vi "DCM System Status.vi"(9 "FIFO Indexes":T4={"System ADC"={"AI 1 [V]"=0, "AI 2 [V]"=0, "AI 3 [V]"=0, "AI 4 [V]"=0, "AI 5 [V]"=0, "AI 6 [V]"=0, "AI 7 [V]"=0, "AI 8 [V]"=0, "AI 9 [V]"=0, "AI 10 [V]"=0, "AI 11 [V]"=0, "AI 12 [V]"=0, "Temp HH 1-6 [C]"=0, "Temp HH 7-12 [C]"=0, "Temp DI A [C]"=0, "Temp DI Zener A [C]"=0, "Temp DI B [C]"=0, "Temp DI Zener B [C]"=0, "Temp CPU [C]"=0, "Temp Fan Intake [C]"=0, "Temp Secondary A [C]"=0, "Temp Primary A [C]"=0, "Temp Boost B [C]"=0, "Primary Range [V]"=0, "Primary A1A2 [V]"=0, "Primary A3A4 [V]"=0, "Primary B3B4 [V]"=0, "Primary B1B2 [V]"=0, "Secondary A1A2 [V]"=0, "Secondary A3A4 [V]"=0, "Secondary B3B4 [V]"=0, "Secondary B1B2 [V]"=0, "Ext HV A [V]"=0, "Ext HV B [V]"=0, "FET Driver [V]"=0, "Fan [V]"=-1, "Battery [V]"=0, "DRVP [V]"=0, "Key [V]"=0, "DI Zener A [V]"=0, "DI Zener B [V]"=0, "Pump Zener A [V]"=0, "Pump Zener B [V]"=0, "MPRD [V]"=0}, "IO Lock"=0, "HH Mode Config Error"=0, "Fan Speed 1 [RPM]"=0, "Fan Speed 2 [RPM]"=0, "Firmware Major Rev"=0, "Firmware Minor Rev"=0, "Internal Fault"=-1, "Fault Value"=-1}, 10 "System State":T1 {"System ADC"."Fan [V]" format="%#_3p"; "System ADC"."Primary B1B2 [V]" format="%#_3p"; "System ADC"."Primary B3B4 [V]" format="%#_3p"; "System ADC"."Primary A3A4 [V]" format="%#_3p"; "System ADC"."Primary A1A2 [V]" format="%#_3p"; "System ADC"."MPRD [V]" format="%#_3p"; "System ADC"."Ext HV B [V]" format="%#_3p"; "System ADC"."Ext HV A [V]" format="%#_3p"; "System ADC"."Pump Zener B [V]" format="%#_3p"; "System ADC"."Pump Zener A [V]" format="%#_3p"; "System ADC"."DI Zener B [V]" format="%#_3p"; "System ADC"."DI Zener A [V]" format="%#_3p"; "System ADC"."Key [V]" format="%#_3p"; "System ADC"."DRVP [V]" format="%#_3p"; "System ADC"."Battery [V]" format="%#_3p"; "System ADC"."FET Driver [V]" format="%#_3p"; "System ADC"."Secondary B1B2 [V]" format="%#_3p"; "System ADC"."Secondary B3B4 [V]" format="%#_3p"; "System ADC"."Secondary A3A4 [V]" format="%#_3p"; "System ADC"."Secondary A1A2 [V]" format="%#_3p"; "System ADC"."Primary Range [V]" format="%#_3p"; "System ADC"."Temp Boost B [C]" format="%#_3p"; "System ADC"."Temp Primary A [C]" format="%#_3p"; "System ADC"."Temp Secondary A [C]" format="%#_3p"; "System ADC"."Temp Fan Intake [C]" format="%#_3p"; "System ADC"."Temp CPU [C]" format="%#_3p"; "System ADC"."Temp DI Zener B [C]" format="%#_3p"; "System ADC"."Temp DI B [C]" format="%#_3p"; "System ADC"."Temp DI Zener A [C]" format="%#_3p"; "System ADC"."Temp DI A [C]" format="%#_3p"; "System ADC"."Temp HH 7-12 [C]" format="%#_3p"; "System ADC"."Temp HH 1-6 [C]" format="%#_3p"; "System ADC"."AI 12 [V]" format="%#_3p"; "System ADC"."AI 11 [V]" format="%#_3p"; "System ADC"."AI 10 [V]" format="%#_3p"; "System ADC"."AI 9 [V]" format="%#_3p"; "System ADC"."AI 8 [V]" format="%#_3p"; "System ADC"."AI 7 [V]" format="%#_3p"; "System ADC"."AI 6 [V]" format="%#_3p"; "System ADC"."AI 5 [V]" format="%#_3p"; "System ADC"."AI 4 [V]" format="%#_3p"; "System ADC"."AI 3 [V]" format="%#_3p"; "System ADC"."AI 2 [V]" format="%#_3p"; "System ADC"."AI 1 [V]" format="%#_3p"}, 11 "Device Outputs in":dbl[](array[numeric])) -> (3 "Device Outputs out":dbl[](array[numeric]))   [LabVIEW 2016, in "DCM Engine.lvlib"]
uses:
  DCM Engine.lvlib
  Shared/Types/System State Indexes.ctl
  Built/DCM Classes Packed/Pharlap/C/DCM-Classes.lvlibp/DCM/Rev0/RT/System State.ctl
  Built/DCM Classes Packed/Pharlap/C/DCM-Classes.lvlibp/DCM/Rev0/RT/System ADC.ctl
  Built/DCM Classes Packed/Pharlap/C/DCM-Classes.lvlibp/DCM/Rev0/RT/Internal Fault.ctl
  <vilib>/NI Veristand/Custom Device Tools/Custom Device Utility Library/Custom Device Utility Library.lvlib
  DCM Shared.lvlib
  Built/DCM Classes Packed/Pharlap/C/DCM-Classes.lvlibp/DCM/Rev0/RT/DCM - RT.lvclass
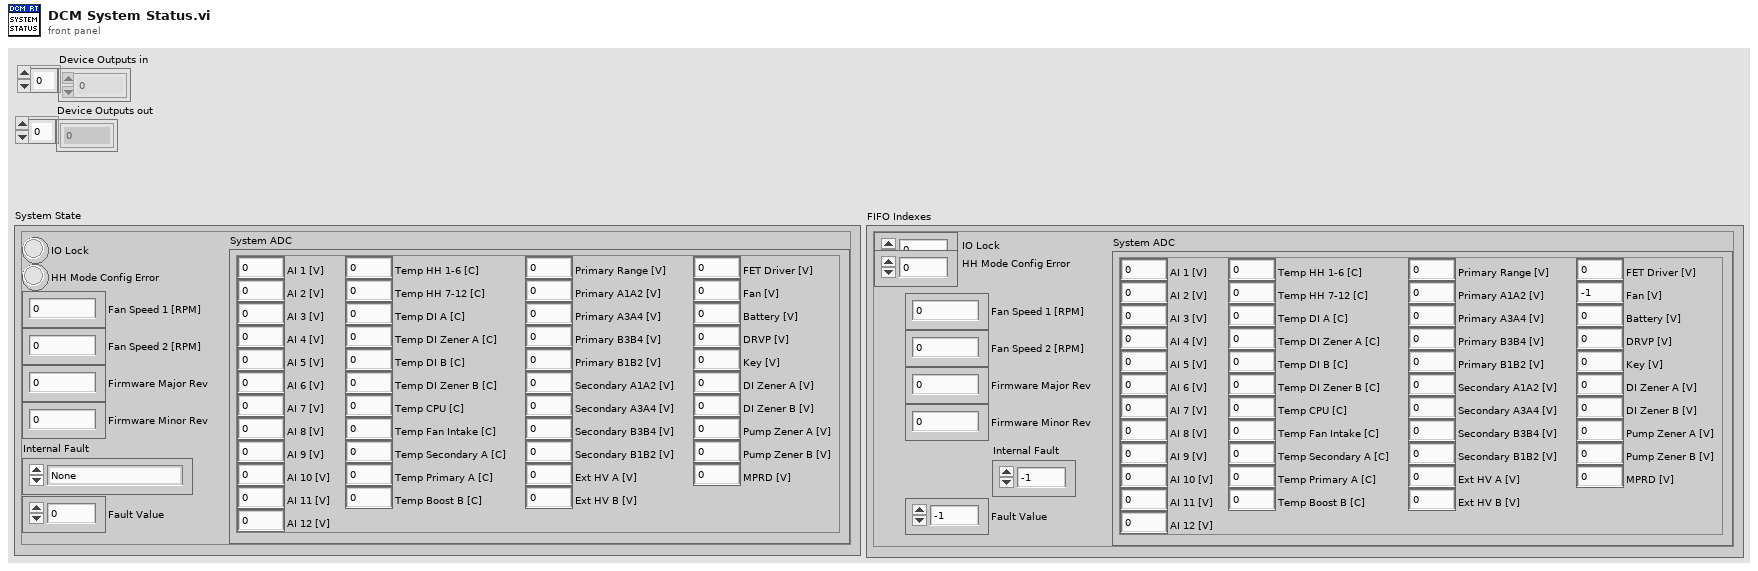
[diagram p1: front panel]
types:
  T1 = typedef "DCM-Classes.lvlibp/DCM - RT.lvclass/System State.ctl" = cluster{"System ADC":T2, "IO Lock":bool, "HH Mode Config Error":bool, "Fan Speed 1 [RPM]":sgl, "Fan Speed 2 [RPM]":sgl, "Firmware Major Rev":u16, "Firmware Minor Rev":u16, "Internal Fault":T3, "Fault Value":dbl}
  T2 = typedef "DCM-Classes.lvlibp/DCM - RT.lvclass/System ADC.ctl" = cluster{"AI 1 [V]":sgl, "AI 2 [V]":sgl, "AI 3 [V]":sgl, "AI 4 [V]":sgl, "AI 5 [V]":sgl, "AI 6 [V]":sgl, "AI 7 [V]":sgl, "AI 8 [V]":sgl, "AI 9 [V]":sgl, "AI 10 [V]":sgl, "AI 11 [V]":sgl, "AI 12 [V]":sgl, "Temp HH 1-6 [C]":sgl, "Temp HH 7-12 [C]":sgl, "Temp DI A [C]":sgl, "Temp DI Zener A [C]":sgl, "Temp DI B [C]":sgl, "Temp DI Zener B [C]":sgl, "Temp CPU [C]":sgl, "Temp Fan Intake [C]":sgl, "Temp Secondary A [C]":sgl, "Temp Primary A [C]":sgl, "Temp Boost B [C]":sgl, "Primary Range [V]":sgl, "Primary A1A2 [V]":sgl, "Primary A3A4 [V]":sgl, "Primary B3B4 [V]":sgl, "Primary B1B2 [V]":sgl, "Secondary A1A2 [V]":sgl, "Secondary A3A4 [V]":sgl, "Secondary B3B4 [V]":sgl, "Secondary B1B2 [V]":sgl, "Ext HV A [V]":sgl, "Ext HV B [V]":sgl, "FET Driver [V]":sgl, "Fan [V]":sgl, "Battery [V]":sgl, "DRVP [V]":sgl, "Key [V]":sgl, "DI Zener A [V]":sgl, "DI Zener B [V]":sgl, "Pump Zener A [V]":sgl, "Pump Zener B [V]":sgl, "MPRD [V]":sgl}
  T3 = typedef "DCM-Classes.lvlibp/DCM - RT.lvclass/Internal Fault.ctl" = enum32{"None", "Temp HH 1-6", "Temp HH 7-12", "Temp DI A", "Temp DI Zener A", "Temp DI B", "Temp DI Zener B", "Temp Intake", "Temp Primary A", "Temp Secondary A", "Temp Boost B", "Temp CPU", "Low Battery", "Inrush Protection", "A Run Enable", "B Run Enable"}
  T4 = typedef "DCM Shared.lvlib/System State Indexes.ctl" = cluster{"System ADC":cluster{"AI 1 [V]":i32, "AI 2 [V]":i32, "AI 3 [V]":i32, "AI 4 [V]":i32, "AI 5 [V]":i32, "AI 6 [V]":i32, "AI 7 [V]":i32, "AI 8 [V]":i32, "AI 9 [V]":i32, "AI 10 [V]":i32, "AI 11 [V]":i32, "AI 12 [V]":i32, "Temp HH 1-6 [C]":i32, "Temp HH 7-12 [C]":i32, "Temp DI A [C]":i32, "Temp DI Zener A [C]":i32, "Temp DI B [C]":i32, "Temp DI Zener B [C]":i32, "Temp CPU [C]":i32, "Temp Fan Intake [C]":i32, "Temp Secondary A [C]":i32, "Temp Primary A [C]":i32, "Temp Boost B [C]":i32, "Primary Range [V]":i32, "Primary A1A2 [V]":i32, "Primary A3A4 [V]":i32, "Primary B3B4 [V]":i32, "Primary B1B2 [V]":i32, "Secondary A1A2 [V]":i32, "Secondary A3A4 [V]":i32, "Secondary B3B4 [V]":i32, "Secondary B1B2 [V]":i32, "Ext HV A [V]":i32, "Ext HV B [V]":i32, "FET Driver [V]":i32, "Fan [V]":i32, "Battery [V]":i32, "DRVP [V]":i32, "Key [V]":i32, "DI Zener A [V]":i32, "DI Zener B [V]":i32, "Pump Zener A [V]":i32, "Pump Zener B [V]":i32, "MPRD [V]":i32}, "IO Lock":i32, "HH Mode Config Error":i32, "Fan Speed 1 [RPM]":i32, "Fan Speed 2 [RPM]":i32, "Firmware Major Rev":i32, "Firmware Minor Rev":i32, "Internal Fault":i32, "Fault Value":i32}
  T5 = cluster{"AI 1 [V]":i32, "AI 2 [V]":i32, "AI 3 [V]":i32, "AI 4 [V]":i32, "AI 5 [V]":i32, "AI 6 [V]":i32, "AI 7 [V]":i32, "AI 8 [V]":i32, "AI 9 [V]":i32, "AI 10 [V]":i32, "AI 11 [V]":i32, "AI 12 [V]":i32, "Temp HH 1-6 [C]":i32, "Temp HH 7-12 [C]":i32, "Temp DI A [C]":i32, "Temp DI Zener A [C]":i32, "Temp DI B [C]":i32, "Temp DI Zener B [C]":i32, "Temp CPU [C]":i32, "Temp Fan Intake [C]":i32, "Temp Secondary A [C]":i32, "Temp Primary A [C]":i32, "Temp Boost B [C]":i32, "Primary Range [V]":i32, "Primary A1A2 [V]":i32, "Primary A3A4 [V]":i32, "Primary B3B4 [V]":i32, "Primary B1B2 [V]":i32, "Secondary A1A2 [V]":i32, "Secondary A3A4 [V]":i32, "Secondary B3B4 [V]":i32, "Secondary B1B2 [V]":i32, "Ext HV A [V]":i32, "Ext HV B [V]":i32, "FET Driver [V]":i32, "Fan [V]":i32, "Battery [V]":i32, "DRVP [V]":i32, "Key [V]":i32, "DI Zener A [V]":i32, "DI Zener B [V]":i32, "Pump Zener A [V]":i32, "Pump Zener B [V]":i32, "MPRD [V]":i32}
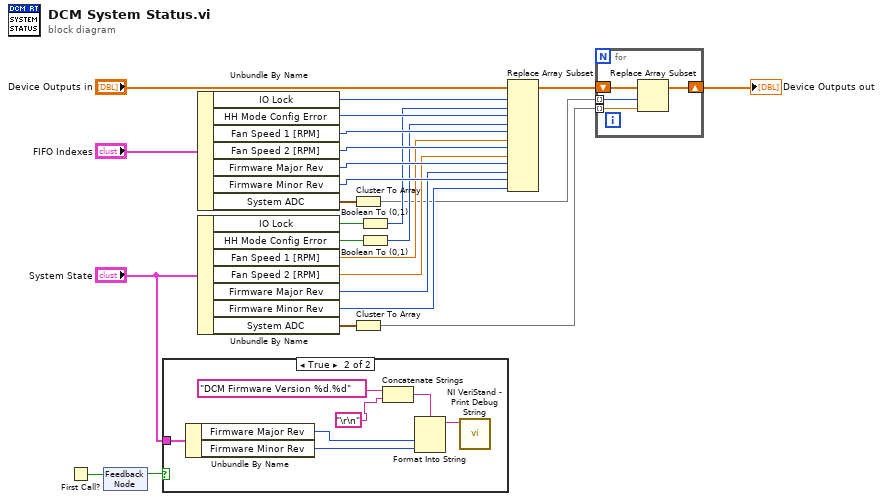
[diagram p0: block diagram]
diagram:
  n1 = First Call?() -> (First Call?: T/F=w1:bool)
  n2 = feedback-in #1(w1) -> ()
  n3 = feedback #1() -> (w2:bool)  [unwired: 1 in]
  n4 = case shown="True" w2 {
    tunnel: "System State" -> [_ w32]
    frame False {
    }
    frame True {
      n5 = Unbundle By Name(w32) -> ("Firmware Major Rev"=w31:u16, "Firmware Minor Rev"=w30:u16)
      n6 = Concatenate Strings("DCM Firmware Version %d.%d" ("format string"), "\r\n") -> (w27:string)
      n7 = Format Into String(format string=w27, w31, w30) -> (resulting string=w29:string)  [unwired: 2 in, 1 out]
      n8 = call <vilib>:"NI VeriStand - Print Debug String.vi"("Message"=w29) -> ()  [unwired: 10 in, 1 out]
    }
  }
  n9 = Unbundle By Name("FIFO Indexes") -> ("IO Lock"=w22:i32, "HH Mode Config Error"=w20:i32, "Fan Speed 1 [RPM]"=w21:i32, "Fan Speed 2 [RPM]"=w17:i32, "Firmware Major Rev"=w19:i32, "Firmware Minor Rev"=w18:i32, "System ADC"=w5:T5)
  n10 = Unbundle By Name("System State") -> ("IO Lock"=w16:bool, "HH Mode Config Error"=w15:bool, "Fan Speed 1 [RPM]"=w12:sgl, "Fan Speed 2 [RPM]"=w11:sgl, "Firmware Major Rev"=w10:u16, "Firmware Minor Rev"=w9:u16, "System ADC"=w4:T2)
  n11 = Cluster To Array(cluster=w5) -> (array=w7:i32[])
  n12 = Cluster To Array(cluster=w4) -> (array=w6:sgl[])
  n13 = Boolean To (0,1)(Boolean=w16) -> (0, 1=w14:i16)
  n14 = Boolean To (0,1)(Boolean=w15) -> (0, 1=w13:i16)
  n15 = Replace Array Subset(array="Device Outputs in", new element #1=w14, index #1=w22, new element #2=w13, index #2=w20, new element #3=w12, index #3=w21, new element #4=w11, index #4=w17, new element #5=w10, index #5=w19, new element #6=w9, index #6=w18) -> (w8:dbl[])
  n16 = for {
    shift-right: [w35] -> w24
    shift-left: w8 -> [w36]
    tunnel: w7 -> [w34] mode=indexing
    tunnel: w6 -> [w33] mode=indexing
    n17 = Replace Array Subset(array=w36, new element=w33, index=w34) -> (w35:dbl[])
  }
  "Device Outputs out" <- w24
